vi "Read Date.vi"(8 "error in (no error)":errorcluster, 11 "Banking Record in":refnum<class "Banking Record.lvclass">) -> (0 "error out":errorcluster, 2 "Date":timestamp, 3 "Banking Record out":refnum<class "Banking Record.lvclass">)   [LabVIEW 2018, in "Banking Record.lvclass"]
uses:
  Banking Record.lvclass
  Banking Record.lvclass/Banking Record.ctl
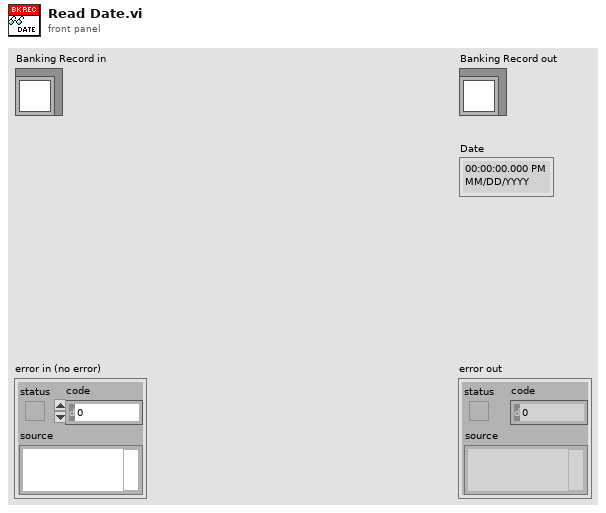
[diagram p1: front panel]
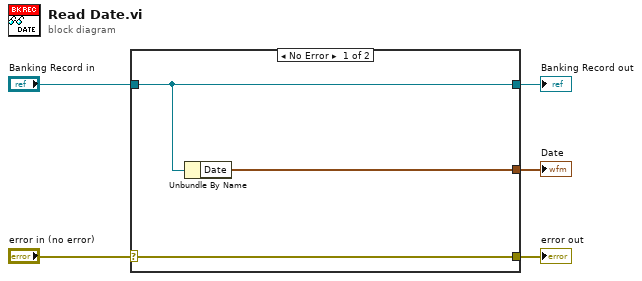
[diagram p0: block diagram]
diagram:
  n1 = case shown="No Error" "error in (no error)" {
    selector: "error in (no error)" -> [w8 w9]
    tunnel: [w8 w9] -> w4
    tunnel: [w7 w10] -> w2
    tunnel: "Banking Record in" -> [w7 w10]
    tunnel: [w6 _] -> w1
    frame No Error {
      n2 = Unbundle By Name(w7) -> ("Date"=w6:timestamp)
    }
    frame Error {
    }
  }
  "error out" <- w4
  "Banking Record out" <- w2
  "Date" <- w1
